vi "TDT ET-Get Event Times.vi"(0 "TCP":T1, 7 "Timeout (ms)":i32=2000, 11 "error in (no error)":errorcluster) -> (4 "Events":dbl[][](array[numeric]), 8 "Num Events":i32, 15 "error out":errorcluster)   [LabVIEW 2020]
uses:
  TCP VIs/TCP Params.ctl
panel:
  out "return value":i32
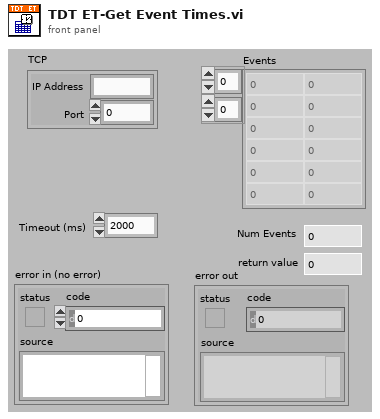
[diagram p1: front panel]
types:
  T1 = typedef "TCP Params.ctl" = cluster{"IP Address":string, "Port":i32}
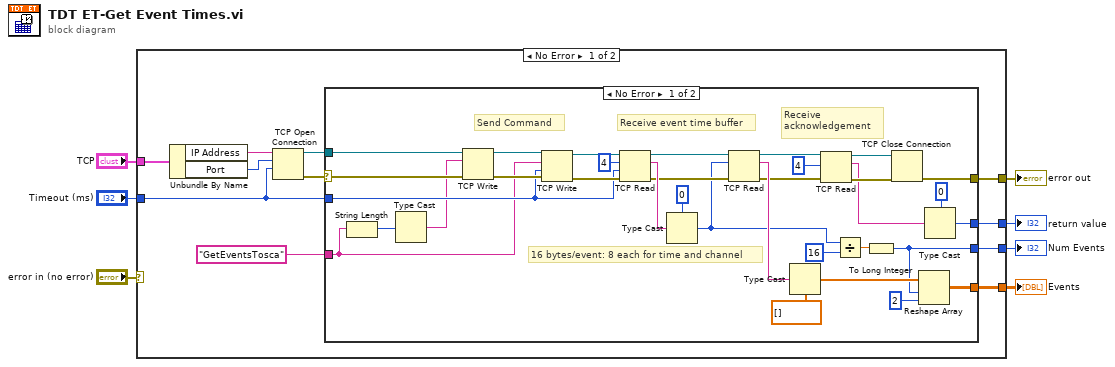
[diagram p0: block diagram]
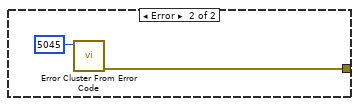
[diagram p2: hidden frame]
diagram:
  n1 = case shown="No Error" "error in (no error)" {
    selector: "error in (no error)" -> [_ w54]
    tunnel: [w12 w54] -> w6
    tunnel: "TCP" -> [w18 _]
    tunnel: "Timeout (ms)" -> [w13 _]
    tunnel: [w10 _] -> w3
    tunnel: [w9 _] -> w2
    tunnel: [w8 _] -> w1
    frame No Error {
      n2 = Unbundle By Name(w18) -> ("IP Address"=w11:string, "Port"=w17:i32)
      n3 = TCP Open Connection(address=w11, remote port or service name=w17, timeout ms (60000)=w13) -> (connection ID=w15:refnum<k5>, error out=w16:errorcluster)  [unwired: 2 in]
      n4 = case shown="No Error" w16 {
        selector: w16 -> [w43 _]
        tunnel: w15 -> [w42 _]
        tunnel: "GetEventsTosca" -> [w40 _]
        tunnel: w13 -> [w47 _]
        tunnel: [w46 w53] -> w12
        tunnel: [w27 _] -> w10
        tunnel: [w28 _] -> w9
        tunnel: [w19 _] -> w8
        frame No Error {
          # "16 bytes/event: 8 each for time and channel"
          # "Receive event time buffer"
          # "Send Command"
          # "Receive\nacknowledgement"
          n5 = String Length(string=w40) -> (length=w39:i32)
          n6 = Type Cast(x=w39) -> (*(type *) &x=w38:string)  [unwired: 1 in]
          n7 = TCP Write(connection ID=w42, data in=w38, error in (no error)=w43) -> (connection ID out=w41:refnum<k5>, error out=w51:errorcluster)  [unwired: 1 in, 1 out]
          n8 = TCP Write(connection ID=w41, data in=w40, error in (no error)=w51, 9:w47) -> (connection ID out=w49:refnum<k5>, error out=w50:errorcluster)  [unwired: 1 out]
          n9 = TCP Read(connection ID=w49, bytes to read=4, error in (no error)=w50, 9:w47) -> (connection ID out=w36:refnum<k5>, data out=w45:string, error out=w37:errorcluster)  [unwired: 1 in]
          n10 = Type Cast(type=0, x=w45) -> (*(type *) &x=w31:i32)
          n11 = TCP Read(connection ID=w36, bytes to read=w31, error in (no error)=w37) -> (connection ID out=w22:refnum<k5>, data out=w35:string, error out=w24:errorcluster)  [unwired: 2 in]
          n12 = Type Cast(type=dbl[] [], x=w35) -> (*(type *) &x=w33:dbl[])
          n13 = TCP Read(connection ID=w22, bytes to read=4, error in (no error)=w24) -> (connection ID out=w21:refnum<k5>, data out=w20:string, error out=w23:errorcluster)  [unwired: 2 in]
          n14 = Divide(x=w31, y=16) -> (x/y=w29:dbl)
          n15 = To Long Integer(number=w29) -> (32bit integer=w27:i32)
          n16 = TCP Close Connection(connection ID=w21, error in (no error)=w23) -> (error out=w46:errorcluster)  [unwired: 1 in, 1 out]
          n17 = Reshape Array(w33, w27, 2 ("dimension size")) -> (w28:dbl[][])
          n18 = Type Cast(type=0, x=w20) -> (*(type *) &x=w19:i32)
        }
        frame Error {
          n19 = call <vilib>:"Error Cluster From Error Code.vi"("error code (0)"=5045) -> ("error out"=w53:errorcluster)  [unwired: 8 in]
        }
      }
    }
    frame Error {
    }
  }
  "error out" <- w6
  "Num Events" <- w3
  "Events" <- w2
  "return value" <- w1
